vi "Time Display.vi"(0 "RedPitaya connection in":refnum<k5>, 2 "Time Offset":dbl, 3 "Time Scale":dbl, 5 "error in":errorcluster, 12 "timeout ms (2000)":i32) -> (14 "RedPitaya connection out":refnum<k5>, 19 "error out":errorcluster)   [LabVIEW 8.6]
doc: "Sets time offset and scale"
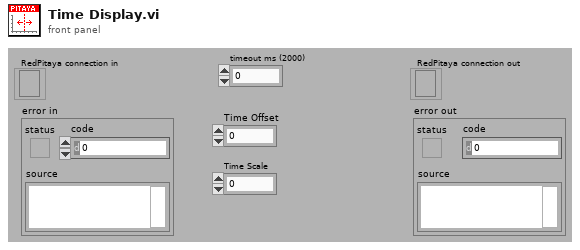
[diagram p1: front panel]
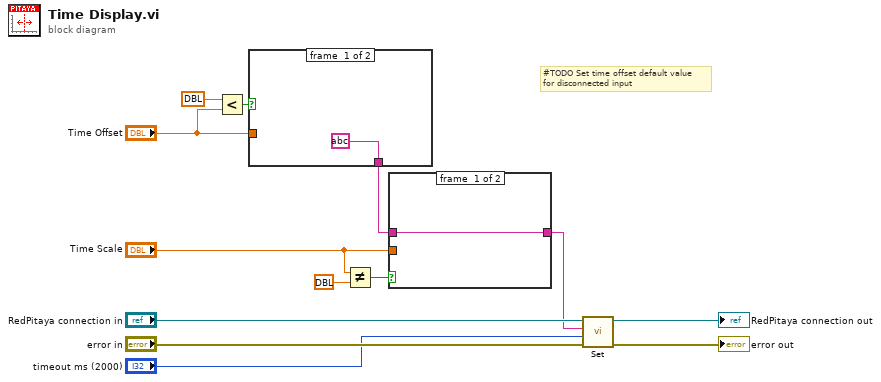
[diagram p0: block diagram]
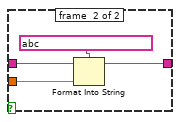
[diagram p2: hidden frame]
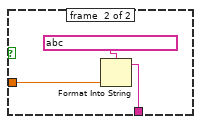
[diagram p3: hidden frame]
diagram:
  # "#TODO Set time offset default value\nfor disconnected input"
  n1 = Less?(x=dbl ?, y="Time Offset") -> (x < y?=w7:bool)
  n2 = case shown="True" w7 {
    tunnel: "Time Offset" -> [_ w15]
    tunnel: [string ? w16] -> w9
    frame #0 {
    }
    frame #1 {
      n3 = Format Into String(format string=string ?, w15) -> (resulting string=w16:string)  [unwired: 2 in, 1 out]
    }
  }
  n4 = Not Equal?(x="Time Scale", y=dbl ?) -> (x != y?=w4:bool)
  n5 = case shown="True" w4 {
    tunnel: w9 -> [w18 w22]
    tunnel: "Time Scale" -> [_ w19]
    tunnel: [w18 w20] -> w8
    frame #0 {
    }
    frame #1 {
      n6 = Format Into String(format string=string ?, initial string=w22, w19) -> (resulting string=w20:string)  [unwired: 1 in, 1 out]
    }
  }
  n7 = call "Set.vi"("error in"="error in", "timeout ms (2000)"="timeout ms (2000)", "SCPI Message"=w8, "RedPitaya connection in"="RedPitaya connection in") -> ("error out"=→"error out":errorcluster, "RedPitaya connection out"=→"RedPitaya connection out":refnum<k5>)  [unwired: 5 in, 1 out]
